vi "Main_19A.vi"() -> ()   [LabVIEW 2024]
uses:
  ENUM_Stripe Select.ctl
  Utility/Universal Utility/TypeDefs_Utility/Cluster_Row-Column.ctl
  9e3f57c0-2ef8-4495-8287-c6a42a5fb955.vi
  Utility/Universal Utility/TypeDefs_Utility/ENUM_4 Directions U-D-L-R.ctl
  Utility/Universal Utility/TypeDefs_Utility/ENUM_8 Directions U-D-L-R.ctl
panel:
  out "Array":cluster{"Numeric":i32, "Array":T1[]}[](array[cluster])
  out "string array 2":string[](array[string])
  out "string array":string[](array[string])
  in  "Select Data":enum32{"Example", "Puzzle"}(tab)
  in  "Example":string="r, wr, b, g, bwu, rb, gb, br\n\nbrwrr\nbggr\ngbbr\nrrbgbr\nubwu\nbwurrg\nbrgr\nbbrgwb"
  in  "Puzzle":string="wwubu, guw, uguggg, bgr, rgbrg, bbrb, rwgru, bwgr, uwwbuw, rwrbrgb, ggbrbuur, bb, ugu, grurrr, gbwbwb, rgbrb, bgrwrbu, bgb, wrwu, rwwr, wubr, bug, wu, brwu, w, grbw, uwbgg, gggwrggb, rurgr, uuw, bbw, wbg, bgw, ugw, brb, uww, buww, uuwgr, buu, rrbugw, ggggbgug, wwwrbbr, rgbbr, ugrr, wgwrg, bwuubub, uugg, bbrgg, bbugw, wuuwb, uwr, bugww, rwrrbbr, ugwrrrb, ubbr, rrwbgg, wb, wgr, gbrb, gwgg, rbg, bub, brg, bubr, ugggw, uuugbbb, grbug, rbww, rg, wgwwwwg, wgb, brugbbb, wgrww, bbrgrurg, ruu, brr, grgwg, wurbb, bww, ubwgr, bburwurb, urrrrbb, rgg, wwww, gbgw, rbrb, buw, wur, ruugugb, uwugg, rgrrugub, ggg, ggr, wrurr, bgg, uuru, brbg, rrbb, bbr, gbbu, grug, rwrrug, ggubub, ggrgg, uu, grb, rrrwwbg, ubbg, wgwwrgbr, rbug, rwrgwbrb, wubwgu, rrw, ruw, rbwubwgr, wwugg, bbbu, wgwr, rwgb, ruwg, rrrb, ubw, rwgw, wbr, uwgrb, rbwrrrru, guwbwg, rgbwr, wbu, ubgu, uruug, urbuuruw, rug, wg, gugbw, brw, wgrb, rbwu, wrw, bgggr, rubu, ur, uggrur, ggwbbuwu, gggr, gwu, bbwb, rrru, rubgb, wub, rgb, rbur, wuwbb, rbb, bwb, wwr, wubrwb, bwwwg, wwbwww, ugrrurw, grg, gwuw, uwwww, ubgb, gwr, gwuurgg, grwuu, gbru, rbbrrg, r, rgbrrg, ugrrubr, bw, wwbwbg, brbwbwr, rrrbg, rggb, bgwu, rrgrwwb, wrgrrb, grw, ubu, wgrugw, bbrugug, wubuwrb, gbrr, rrbg, bbg, bgrwg, urwu, uug, gruruwb, bur, rbwrguw, gbbuw, wubbr, gwurrw, rurr, gwrubb, wwwrw, wrwrbbr, ubbru, gbr, rwg, rrgwgr, ugrwwg, wwbgbr, wwubuwu, uwbb, gggbb, bru, uwb, bgru, wgu, gbrgr, urrwb, ub, u, bgrug, rrwr, bguug, gwbb, uuu, brubwg, bwrwbu, ruggur, gggww, rgu, ug, gur, wgurgwb, uuwwb, wbwgr, gbrg, rru, uuwurrr, rbgbw, ubgwgw, wgwbgu, brbwgg, uwwgw, rgww, buuu, uwu, wrgug, gug, rr, gggwb, bgu, grwg, wrwr, uub, gbuwwrwr, bgug, bwg, ubg, urrb, bbgggw, uuurb, ggw, wgrbwrg, bguw, brrrb, gwrbr, brbw, ggrrbu, uru, wrrbg, ubr, ggrr, ww, wwbgwwr, bgrr, wugbrwg, rrrrg, rww, wrbg, ubur, gwb, rgw, bubgbw, gbb, buuuuur, wwu, uubwww, buwg, ugbg, wgrwbub, wurwuu, bbu, wuru, ggu, wguwgr, gbw, gub, grr, rubgw, urrurb, wbubrr, grgwwb, gbwwru, urb, ruuw, urr, gu, bwrbwg, wrr, wru, wug, wbuwwwwg, guugu, brwurrb, brruuw, wuuuu, rbu, gwg, bgwg, rgr, bbrw, bu, gbbg, bbub, bwr, buur, wrgg, wwuurbug, bgbu, ruburubr, bwurbr, rbr, wgw, gwwug, rruu, wubgg, bwwg, wgwbwu, gwrr, wbbrrb, rwbgbbbr, gr, rwuw, rggbur, gbu, uggb, gwgr, guggbuu, gugw, brgww, wuw, rbubgbu, wgwbrb, g, urbb, gb, gbwu, uuug, ggrbbw, wbrrww, wbw, ugb, gbg, ugr, ggwww, rwr, rbrbw, wrg, wwbr, uggu, rrg, gwguuuuu, bbwuur, rgru, bburww, bbbg, wbb, uuugww, bwgg, bgggw, rugbr, wugrbwr, urw, bwu, uur, gggwrw, buwr, rrr, wwb, wgbw, urg, uwgbw, gru, bgbgurw, rwrrgbub, rwrw, buuug, wggbrgw, guu, bruuubw, gw, wuu, rrb, uuuwg, uwbugu, ugbbrr, wr, uw, ruwbw, wwg, ubru, guub, wrrwg, www, bbuuuw, guruub, wwbrwu, rwgbuu, rguruww, bgggrwr, bg, uwuwr, ugwub, ubgbu, ubbur, rub, gww, rw, urrbbbbu, urrbb, wuwu, ubuggww, bbbwg, ubugg, grgb, rwu, rugbug, ugg, wgg, gg, ru, wruw, wrrwuw, rubg, rbw, rwgwr, uuruu, ubb, ggb\n\nuwgwguuguruwggwbrbwurruwgwwwurgbgwggwwbbubgugguuurgugugwu\ngwwggrgbwbbguwgbguubbwrbgurgbburrgbwruwgurgwgguwbwgbgrr\nrgggbwgwgwuubwbwrrbrrrurwuwurgubuwrbwrbbbbr\nrguruururrwbbrgrbgrbwggrubbggbrbrugrgugggurubrbuuw\nrruggbrruruggubguwrubwbwuwgrwrguuurbrrbbbggbrwg\nwbwurbbrggubugbrgrrbuuwubwurrwururgbgbwurubbuuwbuw\nbrbwrrruwrrrubrwuugrbuuwuuwrwrbrrgububwurugbwwrb\nrbbbuurubwubbuguggrgwgwgurburugugwbgbuwbwwrrgugg\nwrbbugrwgwubgugwrruggwwggurrwuugrwrwbrwgrww\ngbwbugwgrubbbbburrbwugbwuugrbbwrrwbgrwubgwgbbb\nurgrwbruurbbururwrwwbbubgwbwurbwguguwgrbrgugugwrburb\nwubuubwggrgwgbgububrwgwbbubgwgbwwwuubrbbbuwbr\nwrrrrurbwubwuuggwguuwwwububrwrruwurrbbbuubggwgrgwugwu\nbrurwwrbbuwgugbruurgrrgbuuwrbwrugurrwrurrrbbwrwbrrgrwuwg\nurgwuwwbwwrbbwbwgwgrrbrwgubbrbgwububbwurggbrgrggbrggrrrwgg\nuugwrbwguuwwgbwwwburburbwburwgwguwggwggwbbbuburrubgbbguugg\nwbwbguuuuubwwbwgrwbwgguguwgbbggwwwurgrwgrgbgggurbuwugwrbu\nuubwuwuuwggbbruwuwbwbgwbwrrguwurubbguwwgbug\nbwwgwwubbrrrrwuubwbwrruurrwwwwggbgbrwububwwurbggwuwbgu\nbruwgrwwbrwbgruubwbbbugwrbbgwguuwguurbrwrb\ngrbgwuwwrbgrwgrwurrwbbuwwwwwbrbburrbrwbuggrgwbwrb\nwgggrubbbwwgwgggwruururugbrguburrwuwwurgggubrbwwgrwrb\nwurbwrwwugrgrgruruuggbbggubwrurbrgrbwwrbrrw\nuubuwwurrrrurubbbrrugugubgbruubbrwbuwugrwwgwrrbrwggwrb\nggbuwrwwwbbrgruugrrbrbuurwgurwgubrggguwbubrrbbwgwrb\nugwgurwrwwbrrbwrrrruwbgrwrurrrrrgugurwbuuubbubwwbgrrrbwrb\nurwrbbrbwgurbuwrgrurgwggubbwubuggrgbuwgurbbwwbbwwubwrurgrw\nbbugbwrwrrrwbgugbgguuwwbrwbbwgurubrgugrgwurrbb\nuburggbrbuurrbbggububwbuuubgwrruugbrrbuuwb\nrrwuwubggwrwruwrgrrwrwubwwrbbbuggbrggurubwubwbuggwu\nrwwuuubguwgwuwgwwwggwbwrubbrguuubrurbwuggubwbruwrb\nruugbuurwwwwrwuwurrrbrubugubwrwwwgbwbrbgbwb\nwrurbuuruwrbwgrbgbbwgwrwrrrwgwrurbrbuwrwwgbgwgrwgu\nbbruguugubrrgrgurwwggwurwbgwbwbbuugwwrbwubwgrwrb\nbbwgrrugwgrbgwbbugugwuubrbrbrbbrrrggurgbbwwuwrbbuwbgw\nrbgbwburggggrbwubbrrrrggbuwbguggrrbuwbgugbbrgwrb\nubgwuwbbgbubrgbububwuwbbbburwurbwbbuburwrb\nbbgubwgruwbuwbwrwrurbrbrubuwbgrugwbbggbwgrwrburguggwwg\nuwuubwuwgbuurbugubbgguburbugugrrwbrrurgwrwgrgbb\nwwuuugrwuwurbgwwbrbwguwugbgrbgwwbgrgbubrrgrbbgwrggwgrwgruu\nbbbwurgwwbwurwubbugrwbwbgbwrbwrwububbgbgurwwruwrwrrggrugr\nbubuwbbwrgrwuggbgrgwbbwruubggubuwguwgrbrrguwgwubbbbubugw\nwbwbguwgbrgwgwrrurwwrrrgbrwubrgwbwguwbwwuwgugwgrbbubgru\nbwbrbwbrbubbwwbgwwuwgwwgggrrgwbubbubwwwugrgwgr\nwgwwwwurwubuugruwbrrguwgubwwbuuwruugbwrubr\nrgbbbwrgburwuwwbwubwruubgguwbrbwbwrwurbggbwbrugwgrubrgbbur\ngguwwggubgrgrgrwuubruuurubrbrruwgrrwrwuwgrwwburwuwrg\nuwbgrrwbbggrwwgguwbbgbbrugruugbgrbuwgbugwrb\nguurgurbwbbrugrbuugbgruwgburwrwwrbgbrrrgbwbuwrb\nuuwuggwrwgbgbuguruwrgbrbrubgrgugwbrugwrgubbrwuwrb\nrwgguuubwrbbrbubbgwwgrgbbrrrgggbururgwgbwgugwgbgbrbbb\ngrwwrwbbruwubgbwuuubwgubguruugubbwggrgurrbwurgubbggwb\nbwuwbggbwbgwbruuggruurrwrwgubbwrrubrwwbgubguwrb\nrbwbbrgrwgbgwgbwrrurgbrwgwurrwbrwwuwrgugrbgrugrgubbwrb\nwbbgwgbwrubuwgurwbwbugwguwwwgbuwgruguwbgbgbuubwuwgwubgrbww\nuwwbwrbubgbwwuwwubbgbgubwwwgwugrgugrwwwgwbubrguggbrgrbrgg\nwbwuwgrwwguwgurwwurwubgwuwugrbbggbrruuwbgurrru\ngbugwgrurugwrrggbrbubrugggwggbubwbwrubububgbwrgwuurugwrb\ngugrgwugubwuwbbbuurrwwrubbwwwguguwwbbruuugbrwwwuwuw\nrwbbgbugrgburrggrgwgubggwwruuggubururggrbwrb\nrgggggrbbrgrrugwwwgwbwbbrrbrburbwbwwrrgrbuugrruwbbuwrb\nubbuurgrwwwuwbwwbgguurbbbgwbuugwgwuggrrbugguruwwrgbgggbbuwrb\nbwuruwwubgubbggrruwgbbgggwrruubgurbrbuuubrgbwub\nrbubbggrbwbgwwrrbbggubwwurwgrgwubgrgrrbwrb\ngwwbgwubrububgwrurwgurbbuuubwugggbrrwuuwru\nwguggrbbbwgrbrwwggrurwbggwgbrgggrwggugbrgwgg\nuuguuwwrguwrrggugbwwgwuwrguwbguwuurbwbwrggwguwrubwrb\nruuubbgrgrrrgbbrbgbrbubgbubwguububuugubgrugbgrgwrgwrwruggw\nruurrbwrbgubbuwggguwbwububrbwgrubbwgugwrb\nbbgbugbrubwggbrrwwuwrwwwwrwbgbbggrrwbguwrbwrb\nbrbugwrwrbwwwguwrgrrrggugwwruwburugurrgrurbguwguwwbrubu\nwbwubgbubwwgrrggrbbgwruwrrugwwrwuuggbuuwburbrugbguwrwrb\nuugbuuwwburgbgruuruguuuwrbwurwggbbwrrbgrurbwub\ngrrwguwurwwuwgguuugurwrgurrwgrgugrurururwrb\nwwrbuwwwwrbbgwgwbgrurburbbwbgwuugbuwuuwwuuwbbuww\ngggrbrwrugrrurwugwgbgugrruwrrruurbwuubbuuruuub\nrwuguwurugbrububbrggrwrwururwuwuwbrwwgurwgrrrrbrururrwbgbwrb\nrwbbgrbbwgbrbbgugggwwububugrbrgwgubbggwgrgrbrrbrgwwuwg\nwururwgrruuwrgrrrwbruubuuwgbrrwbgrrbbbgugbgrrguugwg\nuruwurbgrwrgwbrbbggwwbgwbgwrbrgrrugwbwrwwbggbrgrugwrb\nwrubuwbugurguuurugburubbrgrurgwugwwbbwuwrb\nbwrwgbwwbuuwbwgbwbbbrbwgwrugbubbgubuwrrwguurgrurwwwbwrb\nrrwuuwbruwugwguurgubwrgwgwgburbrwwwgbubwrwrgggrwugurbrrbu\nrrwgrgwwubwgwbrubwurbbrgbuguwbuggbrwrururrubbwburw\nuubrgrrbgguggwrbwbwwwguwugugbbuubgugrrbugbruggrwubu\nuwrrubgbrrgrbgrrrgbrwgwgrwbwgugguwwwgruwbuwwrb\nwbgubgrbrrrwbgrbrwrggugruuguugubbwrrwugbbrubrrbuubbwrbwrgw\ngubggguubrrguwrwurubwwubbugrwugwugguugguugbuwwwwubgwgbwwuu\ngwguwggwgwbrugwbgbgruwbrwgbgrwbgubbbgwgwbggrw\nwwwburgwwurgubugwrubrggbgbrrbgbwgggwrggbwbbbbubrbuuw\ngggggubgburbgrguurbruuruguwubrrrbruruuguwwwgggu\nbggruubuugbbubugwrrbuuwrguggrwrwurubgbwwwbuuuwgubguruw\ngwgbrgburrbbgrwgrurguuwrrwgggrbgbbgwbbbwrgggwbrbrgwur\nwbbbbrggurwuugbruubrbwgwgurbwuwbrbwrbwgruwrwwgrwurwuruwrb\nbbggrguugwrguwbgruwrwbggurbguuuubgrurwbbgurrbgguggubw\nuwrrwbwubbgwbuwwuwurgwurbrruruwuwguggrwbwwurwwurgbgu\nubuubuwrgrwugguuubwwgwrruwwbuwggbbwwrrwbrgbuugugwwr\nrwwbbugwrwggwwwuwwbgwwrrrbggruruburubrrubggrgwrb\nbbgbrwgwrgguwwrubgwbgubuuurbwwbbbbuggbrgbwrb\nubugbuwbrguwwbrgwrgguwwburgbuubwwgbgrbrubgbgr\nrubwrrgurbuwbrggwgbgwbggwuwrbuwgbgubrrrgrrwgbbg\nubrbrrgurwbgbbbrrrugbrwwgwugbrgbugugugrbbggrwbgubbbuuub\nwuwgububguurguugwuwbuwubgruwbwuwbubuwburbgg\nwwrbgwrgwubwrgruuggwbwwbrbggurburgrggubgwrrgrgrgbbrbgwwuuwrb\ngbgrrbugugwrrbuwrubwuwwgggwrbwwrugbgbgrgrrruw\nbwwgwruwugwrgwwburrwrgwgubbrgurgubrwwrggrggbwwgrguuwww\nrbbwurrgrwrbuwruwuwuuwrgugbwrgrgruubwburbrgbrubgrgrwguur\ngwwuurbugbgwuggwwwwwbwgrrbbgrgwwbwgrggrwrbugwrwrb\nugwrbrgrggwbwwuubrwubuuwwurbbbbwgggwgurbggw\nbbwggbubgwwuurbuguruwwbgggurgwbgrgrggwurrrrurgbrrugrgwgww\nuugwuwubrurururbggrrgurwgwgrrgwwgrwurwrwurwgruu\nuwgbwurruruwwuwgbbgwwrrwrwbwgrrbwbrwgwbbwubrgruwub\nguugbrrubwbrbgwrwwrurrwwgbbgwgwrbuggurgruuwgrub\ngbgurwuuwubrrugwrrugwbbbrwbrwuggrwrrugrwbgu\nbwguugwwwuruguwrrwwbbuguugbggbwbubbwgwrgbbguguruwguwuru\nbbwrbrguwrwbrgruguuggbgrbrruguubbuwwgrbbuwrwwgrbwb\nbuwbwbbrurrbubrwgrgwwwbgburbruruwbbbubwrbuuwgwwbwu\nurgrrrurgwrggugwbrwubgguguuruurubbwrrrwrb\nbburwruuwbugrbwruuuwguubrbuwuwbgbgrbubuwbgr\nrbgrugguurbrrbbwruuuuwgwrggwwurbbrggwrruuuurgggbrbrbrb\nrguwurugbwbwrbbggrgbgrgbwwuwrbbubugrwrgrrrbbbrburgubgurggwrb\ngwuwuuwugwgguubruwwrubrurwrgwrbbgruuuubwwurrugwuuugwubg\nbgubgwwbrbrwruugbbbbbwrbguwbgwgubgbbgbbgurgrurgggugbbwbr\ngruwwbwwgbbwwbwgwgwwubwwbwubwrwrgurwuwgrbbrurgwg\nguguwggbbbgbggbrbrgwbgbrwbgrgruurwurbwggbuwug\nrbrbbuurgbgbgbgggbrrwuwuwgwbwbwwuwbgubbbbwr\nbgbuwugbugrwwwwgrbbgguwbrbwuuwgrgggrrbgwbwgruggggwwubbwrb\nggwuurgbwurbwubbrgbbubgrwguwbrwbrruwgwgbrwgrrurggwub\ngggruuubuwrrugggruuguubbrbbgbruubuwrurwbrwggbrgrrburwggw\nrrugwrwbrgbbwrgwgbbbrwrgbburubggugrwggrbrbwubrgurgbwrb\ngrbrubguwruuwggbwugwwgwuwwggubuwuwwrggbrbuurwubwbbwrb\nuwbwuwwbbrguburrwrugburgrwuruwugbburubwguugwwru\nuuwwrubggwwwuugrgwbwgbbwrrbburuguurbrbwuwwrbggurbbwguuw\nubugbwrguwrrwurwuwbrbbubbbwbgugwgbrbwruwwwrububgur\nggrrburgrgburuwrrubububrrbgruuguuuwwwgwwrgbruub\nggbuugwurgbgrwggurugubwggbbbubrgurrwwburuggrrrgbbbbwg\nggbrgrwuuwwbwbuwwwwgguwbbuwuwuwuwrwgwwubwwuwrb\nwrbrgugwrbwrwguggrrggbguwrguuwbwwrrubgbbbuwwrrbrg\ngbwbwrgrbwurwuggwwrwwgwrbbwrwwrbrrrrbuwuurrburruu\nbgugggbbburbbbrguurbgrugwwgggurugbuubuugubwrwr\nwrgbrrrbwwurbgbgbwbuuwbwwbugbgbugrwgwuuubugwrggwwbbbwggwgwrb\nwwbwbbrwrbruwrurwurwggwwbrbuugbugbrwgubggrr\nbrbubbburuwgrbuwwuwrurrwwubrwugwbgburgwrggbwuwrguwgwuu\nrwurrbrggrrgbbgbuububrrwbguwrgbwruwgrrruburuurwwrwbuwgbbr\nbwggbuggrwuubrrwubuwrgwrbuwwurugrbbguuwrrugbgburggububww\ngruuwburbbgbrbwgugwgwuurgububuwugguwuwwrbw\ngrrbgwbwrbrwgwrwuugwbbgrrggggwuwgwugbbgugwbrugwbwu\nrugruggwruburugwugrgwbugwwugwuwrrgrgrggubrgbwgwwwg\nurubrbgbgrgwwgwbrgbbwbrruuruuruuururggubwr\nburbwguggwrggrwggubuurrgwbgwggwrugwwuubgrbwbgrrbug\nwwbwgrrwbwwbrugrbgwgwgrwwggwbrbwbgggguuubwbgbburguggub\nurrbbbburgwbwbbwrgubbggrwbbubuwrgggubggwrb\nggugrbggurrbggrwruwgrbrwgwbuurrgrwwwgugurrrbwgbbrbbggwrb\nbwgubwruwrgbrbwgbwbbgbwbgrbbruubbuugwburwrb\ngwrbbrwugurrbugrbgruwruwrwwguwubwubwbrwgrruggrr\nrwgubrrugrwwwubrwwwrbrwwrbgruwgrubbgwgrwrb\nbrrbwgwgwggugbgrrrrgggubbwwwuururbgbrwugwbrbrbwuuwru\nurbrurgrbgguguguuruwurgugwwgrubggbgbwwwgrbugubwggr\nrbgruguwrurwbgwgurrwrrrggugrwwbrbrbwgubuwubruubwrurrgwbgbwrb\nggbwuuuwggggrububwwrurgbrbrubbwgbbbgbbbgbwuwwgggbwrbuwrb\nrbbbburwggwurrrrbggwgwwrurubwbgbrbruguwwrwrgggrugubw\nrgwgwwrgbrgrwgrrbrburwbwuugbgrwwwggrwrbbwrb\nubgrwwwuubwwwwgbbrurbuuruuurrbuwggbbuurgrrwrgwb\nwgwwuruurbgwruugrwgrbugrbbwbgwwgguubrwrrbr\nbwrwubggwgrrubgrrwuwuuugruuuubuwbrbbwrrbgrwugwgwugrguwrb\nrguwgwugururbwwgwwwgwgwbugubbrbrgwrwgguguwbwruwrrrbgbu\nwuuuugurbwrgbuugbrrwgggwwwrwrrrrgwrwggwrbb\nwwbwbugrwbbuwwwrwrrrubrbgwwwburwgbgbwwbuwrwugguurbg\nubgbuubgrrwruwugwbwbwbwwgbwbuurwwuwbubwrbug\nuubgrgrrugubggggwgrbgbrwrwbrgrwbbwgrburrbr\ngbwwugwbgggrbguurbrburbwwrugguwbugwwugbuwwbguu\nwuwgrgrgwgrbuwgrbgburuuwrbwguuwuruwgbwwubwwbururbw\nwwrwgugurwrbbbrwbwubggguuwrwbuurbwbwubggbbuurrwwbubuwrg\nbburgruburubrbwrwwwbrgrbuwgwrwggurburubrgwgbbruw\nubrwbwubbbbwbwgruwuuwbrgbuwwuwuurrrwrrrwgb\nwwwwrbrrguwugugbgrggrubbrgrurggbgbuwwbrgggwuguwugbrwg\nrbrbbuwrubbbugbgwgurggrgbwrrurbburwrwggruwrubgbgwwuuu\nwuuugbgwgggburrrrgwbubbbgrubbgburwrbugbbwbwggrgrg\nrugwgubuwurrguwbwwurrggrgrurgwbbwbubwwgbgrubruuuwwbu\nbgburwubrrwburrbwgwuwwwwurwuuwbgbgrwggubuwubwwggrwrb\nuurbururruggwrwuwbguwwwbbwrbbwrggwrgbwwugwrwuwrw\nbburugbugwwwwggggwruwwggrwwrbrrbwgbbbuwgwgbwwwubgrgbwrw\nrgggubrrbgugguwwuuwurgubgwrbuwubwburwuubrgb\nrwrgwbrbbwrbuwwuurgwuwwbrbrwuububrgubbrbwrguruuub\nuuugrguwruwwuwuuwgbbrrwwgruuwbbgwguwwruuwrb\nbubbubgwwuurgwrbuuurrwrwwrurwgbwugguwgbbggggww\nuwruwuguubrrbbggbgrbwrwwwbwwwggggruuuguuugbwrwwrgw\ngururwuubwbbugububgwugbugguwuwgwrugbrwrwrb\nwrrbwuuwbwbubgwrruwgguwgrbggubrgbgugrrgrubwwwbwbr\nrbgwbgwububrrrwbuwwwwgrurwrbwrgurwruggguggurrrubbbwrwgww\nwggbrggbrrgbrrgrggwbbwurbbrgugugrbrgrwwbrgubwrwuuruubwugwrb\nrrgbggurbrwuwrgrbbwwubguwgurugurwurwbgwrrbbwwuwwbg\nwbbggrwrgruwgrbrgburwggrrbbbguurgubbuwbruwwrggrbr\nwubugrwrrwuuugwuubgrubbbbgurguwgrwgruwwruguburwuwu\nwbwuggubbrwugwbwrrwurgubuurrrubrgwbruugrgbrrbrugbwrruwuubwrb\nrrbuwruwguburwgugrwgwuguwuubgurggrbuugbuwrb\nwrrbuwggurrggwubgwwuggbwuuwwurrrwwrwurrburgwbwugrgbuwwrwrb\ngrrurwggwgruwrrbbwuugrwgrgggbrgubggbugugrwrb\nwwwrwbuuwgbugbwurrgwuwbuuwrbuurugurwbuuuburrurwrb\nruruggbgwbggrwwrwrbrrgwuguwwrwurrguwugurbbruwbrwuu\nuwuuggwurgbwrrrbruwrrwrurgrwrbrwugrwbbburwurbwbru\nrrbwuwgrwuugwguugbrwgubrbubgguwrugrwbwrrbggbgrrrugrbbgr\nrgggrbugbubburuwwbrrrbuubrrwubuuuwgbgguuuurrubrwwuwwugrbwrb\nurrgwwwrgwrrgurrgwbbrggwrgubwgwwwugruuubuuwggbuur\ngbuguuwwrbggrwrrubwwgrbwrurugrwrguuuugwgwrrrgubgbwb\ngwugrrwrgubuwggwrrguubugwrbururwgbwgbbugwwwrb\nbruuwuwbgrbrwbwwubrbbwrgwubgggwugbuwgbrwbbwruubgwbbrwwwubg\nwwgurbbbbbwbwwrwguwbrururbwurgbgwurrurbgur\nwwrgwuurruwuwugbbrwbwrbbbuwgwwububrwwgggbguwrgwrwrrub\ngugwrrrwugugruuwrguwbwwubbggrwbgbwrugbuwrb\nrgubwgbggwbbwggwgggrrrgggbuwwrgrwggggrrgwr\ngbgrbggbgggggbgugwgubggwrwwwrwgrbrguwuwgwrbbrbuwwgrwuwrb\nwwbgrrggrbgrbwbrrrbwrwrwbwrbrrwbwuugggwrb\nwbbwbwbgrbwwwuguubbwgugrugbbrbbggrwwurururwggw\nuguwrggruugrgwwuubbrbbbgbbgugurruwruwbugwrugubwwbgbwg\nruwbwbrubggruwbrwrurbrrrbgrrwrrgbubbrwrwurwuubwbrruburwuwrb\nugrrbgbbugruruwbgbbbgwbuwgbwugurbrwbgurggbubwwrbb\nwbbwrwrwgurubwgbrgwgrgggrguruubburrubwugggrrwgbbrugw\nuugwubrgwuuwbrrrbgruuwruwwbuuubgwuwwwuwbruguuuwgrbrwrb\ngugubrrggwbuugubrbgwgbubwwgrrurubwwrbbwbrgrr\nwrggwguuguuwbgburwwgwgwbruwrgrrwuwwrgbgugurwggbbg\nwwuugbgggubwwwgrgrbguguwgwwwgbuwgbugwgwwguwrug\nuwuurugbwgbrrbgbbuuwuggbrbrwubwbrggwbgrubbrrggbuubu\ngwggubgwgubguwrbggbwwgbuurbbuubuwwugbubwbgbbruu\nbbubugbuwwgbgubrbrguwggbbugggbuwuubbwgrwgwg\nrrrrwugwuurrrbggrbwbrbrugbrbubugrbubbrguwwwwwrrgwgbuugbu\nwrurguruugbwrwbgguggbwruwgbbwgguurwbgubwruuwru\nrwbbwbrbwuwrubgbgwrbbuwbgubrgbwrrwwuwgbrwgurgubburuug\nggwubrwwuggrrwbuuubwwgbbgwurwgrgwwuwubbrgruurugwuguggurg\nbbrugurbrurbgrbubwurrubbrbbgugwbbbwuuuwrb\nwwgwwbruuuruwggbbwuuuubgwbubrbgwbwwuruuguw\ngburwbwbgrbwbgrugbuwubgrrbrrggbuwwrwrwbguuuu\nuwuwgrbggbrwgwggwwgbrrwburuuguwbbwwwrgurbgurrwgwurguwrbwu\nrbwrbuwrwgbbwwggrbwbwwggrwguwggbwrgbrrubgubgugwbrruwwrb\nbbuggbgbwgwrrrggbubrggrurugubuwbwuguwbugrrggwuwbwrggbwb\nugggrbwgwuubwwggggwuwwwruuugrrguwwbwubrrwugwrrurwgbg\nbwgrgbubgbuurggguubwwrwgbubgrrgrgugwrguwruwbrbwrwbbwbbbb\nwrrrbgrbggruggbbuwwuubrruwgbuuubgwbguurrubbubb\nrbwrrrrubruuwgrgrbgwwwurwurgwbugrbbwwgggugbu\nugbggrgrguwwwggbruuruubwwgbwuggwbrwbwwbrbwubrubgbrrgwuwrwrb\nrwrbrubwbburrurbuwgrrrgurwgrwbrgwgwwrbwgbrwr\nwbwrbruubggrgwbbrbgrbuwwrrrbwwburwgwguubuwguwbrgubbwrbrbwrb\nrgrrbwrgwbbuuuruuwbrubbbuburguuburrbgrwbgruwru\ngwrgrrbubrwgurwgruwguurgruruubgubguggbbwwrb\nwgbbuwurburbwwurgbgbwgggruggwurbwuwbubrwrrwbburbgrwgug\nubugbggwuwguwwwuwugwbwgwwuuuggrrrrubwwubwbwrwrrugwbwrgwuu\nrubggguguuwgbuwggrruwrwrgruruguurrubwuwrgruwwgrrurbwuw\nwurbburwrubbwbwrruwrbrbuuugurbwuwwgrbrbggwwbgugubrrg\ngugruugwruwuwrugbgurguguuwwbbrwrurrgubwbwbrgbwrb\nwugrbrbgwbbuuwrrgrbwgwrruuuubrbruwggurgbrg\nrurwugugguurgubwbuuuurrrwbrrurbwruurwugrubrgubwrub\nrubgwwrrwwwgguuggbwuruwwggbrubwbrwgubrrgrwwbuwggbbburwurbwrb\nwbbbggwuwbwwgguruwguwbugwgruwwrwrgggurwwuwbbwubgu\nbgbwbbwruuugugbrwburuwwrwbbbuggugbwubrrwgwugbwguguuuwru\nrbrwwwwwgbruwguuuuubruuurgbuubrwbrbrwurgburbub\ngrruruwbrwwrbgrgbgrwuwrgwwuwbbwgrrrrrrrrrggbbbwbbbbu\nurrwbbbrwuggrggbgububbrbubuwggwuugwurbbbwbbrwrb\nrwwubggwrrbuurwwrrruuuruwggggwbbuwurrurugg\nbgrbrruwrrgrwbwruwbwbguugbrrggrbgububwbuubrububggugg\nrwruuwbuwruuwrrwgbwwrbwwwbwwrwwuuggbggwbbrbbbwwg\nrrgwrgwubgwrwugbuurgruburburuwwwbwwwwrgwwrgwrgrgg\nwgwrrgwwurrrubwgwrgbrbwgbbubrrrgugwwguubuwrbbb\ngurggwuurwwurwrggugwugrbwubggwwwugrbubwrubbuw\nuruuwurrggwbgrugrrbbubwbwwggbuuugwgrwbuuuugrrwbr\nwbbguguuwuubwwrbrbbrugwrwuuwgrggbbwurrubrrgwwrb\nrruuugbgbgrrwwrwgrbugburbubuuggurguugbwgggwrwwbubb\nbrbgwwbgrugurrgurbbwbrwubbrbrrwugwrwugrwwrb\nbuurubwuubrwbugwbbrrgwbgubrggubwurggwbrwwrrurubwrgrrg\nwbrbrrrgrrbwubwgrwubgrgrwuubbgwwwugbwruwugwwgubww\nuwrgbrubwbuubuurrrbwuguwbggurbubuwgwbwrggbggbwruwuggguwbw\ngwbwgbwbgrwbgbbbrwwggbgrurgrwguwgrbruuwbugwrbuwwbwrb\nguwbwbrwgbgrrrbbrbruwwbbuwwggbwrrbuubugwbrwrb\nwrubrurubbbuguurrbguugwurwuuuwgubrwbbgguwwbbbwwwrbwgwuwgr\nrurgbrrbwwbgwbubuggwugrubbgwwwrubuuwbgwgbgwugrrugrub\nrwugwrwwbuggwbugbbwrbwwruggbgrwuugruurgrbwwbuwwurubgbr\nbwbwuuubbgurgrgrbggrubuuwrugwgwuwggwrggbrbwubwgwguwwrb\nurrgurwuwwggrubgrrwrugbbgbbbgwrguggrbuggrgrgwrb\nwuwurrrrwbwgwwggurwuwbrrgrburggbwgrggbgrbrrggburrggwwrb\nubugrbugubbwgbbbwwgwgwgbguwwbrgbrgwubbwgwwruubgrgrrrb\ngurwwrggbbbburwbgububbrwrggbuwgbwrbrrugburgrgbu\nubgbbrrbubrrubbggrbgwbwrbrwubwuurgwbburwwgr\ngwbrrgwgubbbbrrubwgrguguggwwrbggrwrwuuururwrwguwgrbuwbuuwrb\nggbubbbbwruuggrwwuuwbbwubgbururrggrbbwgwrb\nrgbbrgrwgrruwrwbuurgugbrububrugbgwruwbrurbrwwuwbbrgbbrugr\nurruuurggrwgugbgrwgubrbbbbwuwrrwgrubrurgrbuwrgwu\nbbwwwwrbbuwubgrrgurbbruwrbrwguwrbwrurwwwbbuwgruubwwwrb\nrbrggubbuwguwbggbrrbbwrrurrrbuuuggugububbbbwrrwb\nugwgwwwrwruugwrwrbuggwuuwgbubwgrbrwwgrggrrgrbrbgbbwgwrb\nggugburbbrgrrwgwbwbwruuwugrbrrrurgwrbrrbrwubr\nububbrggggrbruugrubrwrbgbwggwrbrwubggubgggrrgbubrrgrwrb\nrrgwwwrugrurwuggggwrbbwugwwwwububgbrbguwwwguwguwrb\nuuwwwrbgrrbwgwuwrwwwgwwwrbbrbuggwwuguurwgwrb\ngurrrubbgwubwuggrrwwbbubbrgbgubruwrgubggrwgrburrrrg\nuwugubuuwurruwruubgbgbwwggbrwgwgrbbuwugwrb\nwwwrbwrbwwgbrbrwbrggrgwrurrbrbwuruuburbubguwwugggrbwgwgb\nwbgugurgwrrbbwugwbrwuwrwruruwrrugrruugwuggggw\nrwbrwwgrgwwgrwgwbgwrwrwguubuwwbguwggubwggwwbww\nrggrruwggwrrgggbrruwrgbuggbbgbwbwgurwrugwbgwwwr\ngbbwrgwwrwgguurbggrbgbwggbbbuuwururrgrgwgbgg\nwbgruwwwubrbugwbuwuubwgrubguwgwbrubrgwwwgwbgwwrrugbgbub\nugbwugubwgwbuggrurguwwubwrrurrbrgurrbrubwuwrwwwwwgwwgrwwbw\nwrwubuguggbrrbugwbwwwrguuuguubwuruugwbgwbguurgwwbggrwwbuwrb\nuuugbgrgwrugwguuuuurwgggrburwwgbwrurwbgrrwrb\nwbgwguuwbbuwggubrrwbgrgbwuwrgbubruwggbrrubbwg\nubuwbrwbbbwbguuwgugrbuwwrgugwubgrburbgbbrrgrubbbbbu\nugbubrurbgwgwwgrurbwugbwwwbbgbugbbbuggrwgrbugbgwwbuwrbuwrb\nwgrwwuugurbgrrgwwbwrubrgrrwwubgbuggwbbuwubu\ngbuwrwbrrrwrwbwwrgbugrbugbrurrgggrgwgwgrrbgubrr\nwugbuggubuggbrggubwgggbgbgbgurrgwwbrwwwwrb\ngrgugwubbugurgbguwbgbrugwbugbrrwubwrwuwrgbrugrgwrwrb\nguruwwrurwurwugbbrbwwwwubuwrwuuwwugwruwbggbbb\nbguruwbbggggbgugrbgrrrgubbbrubwrrwrwubrwgrurw\nwbbrbbrgbbgguwbruuguwbbbrbrgrubgugwrgbrrgrwruguwrb\nwgrbrgbrgwurggggurwwwggubbggrrrgrubugwuggb\nbbwuwwrwrrubruuggwwbrurbgwururwggwwrrrurrww\nubwuugrgwuuuwururbrguurgrbwwwrrwbwruwrgwururbugrwrru\nrgbbrwbbguggwbrwwbbgrburwbbwwgbrbwbbubwwrb\nuuwuuubgurwwggwwbbbgbgbwbrrgbrrwrbbuwwwgubgggbbrwbrr\ngbuurwggrrggbbrgbuuwrgrggrwgwwrwugugwbgwwbrr\nbwbrgwbrgwwubrgubbbuwbrubwrbgbrrbbbbwrwbgwguuuuubrgrgrw\nguwguururgwuwuuwgwbruguwbbubuwbrggwwugrwruruuugrwrb\ngrgwuuwrbbgrrgggbwrugbgwbbbrwuuwuwgbwugwruurrrbbuggrwwwru\nbuwggggwrrrruburwbrugrwrrgwuguwggwbwbgugrgugwwurbbburrggw\nugrwgbbwwwbbgruubgguuruuuururwwbuugbgwwrgubrrbuwwugggw\nwbrbbugwgburbgrbgrurrbwwwrbwbwubbgrurrurwwrrbwgbugugw\nugugwbwwgrrgrgbuubwrwbrrurrgbubggwrgbugwrgbggubbruubgw\nbwwubbgwwrrwruuruguugugrwgwubbguburuurwguwbwrwrb\nbrrbwugubgwrgurrrgrbbrwrurugrugwuggwrgrbrwggwbbuwurrwwruwrb\nrwbbrbgwgbwguwgbgwurgrbuurugrrgwuwuurubrbgr\nuwwbuuwgbwgggwrububuugrwurgggwgbwbubuurgbwrrwbbrwuruwrrrb\nbbgwbwrrruurwwugbggbbguggguurrbbbbuubbwbwrwbrwurrbuwgrb\ngwgwbwgguwwrwugugwuuwurwgwgbuwgbgbwwuurwwggrubb\nrgburwwwuurrgbuwrgwrbugwwgguwwwgbubuuggrwbgubrwrgwugwbuwb\ngurrbwgburruggbrbuguugbguruwurbuugbrgbguguuuubwggrwgrrwbwwrb\nruggwuwgbgguwwuburgruwrbgbubbwwugrbwuwwbrbrrwbg\nwwbrrgguwbbguubbuuuuugwbbrwrrgrruwrgwwrbbbbwgrgw\nbwbrwbwwrwwuugugugbrbrbrrbwrwrruguwuwwubbugwgurrr\nwggrwwubuwruwgugrguggugwbbggugruuggrwbggrwbbw\ngbgubgbwgurbwrrrgbuwwguwrrwwbwuwuwbgburrbgwbgwr\ngrrububuwruwrubrgwwbrrgrbwugrggwbrgbwwrb\nuguuggrrwubrgrwggububbwgbbwgrwurwwwgwbubbbruggrwbrbgwrb\nbrgurrbwwugubrrgurrbbrbuubbwwwwguwwgrwwugubgruruu\nwrwubrrwburuwbrgwwuggurwrrwbbruruuwuwuwubbubuuu\nbwbugbrrbwugbwrubuwbuwwubbbguwbrgwwurbgugrgrwgwuwwbwubgwrwrb\nbwguwgurgurrrbgbbbwbrrrwuwbrwubruuwrbwrb\nrbubgwbubuwwbubbrgwwgubgwwrrgbubrwbbrwwrbwwuwgbbwrb\nwrbbgwburwwwrgwggggrrbubbggrbgbggwurwruburwubrubrgr\nrggurrwwgururrgrwwwgrugwwbguurbbwbuwrwurrrbrggbbbbrwwr\nugwwgwrgrgugrbbbbubrwrubrbguwbrwubgrwgrrgbgggwugw\nuwgrgbugbwbbggrgrbbgrwrbggrrwbbwbugwrwbrrwwuuwrb\nbguubugwggwguuggbguuwbgwbwruggwrbgbrrbwbrrbgwrbggwrbrrbu\nrgwwbubbbbuugubwbrwuwwrrruuwggrbbrbwguwruuubgbwwgwurbgbubg\nuuwbwbrwwubbrwuuuwuwwgggwwubburgwgwbrurrwbrbgbbburwgb\nwwrrbbwwbruwbgbggbrbbgrugubggwgggugrbuurgrbbgbuwu\nugrbwbwwgggwrgbbguugrgggwrggbuuwuwubrgbruwbwrb\nubggwbwguugbbubbgbbguubwuubrbwubrubrwguwwwrb\nrugburrbwruuwrwwgwrwggrubgwbuuubugbwuurgbg\nggrwrruwggbubrurubgwrbwrgbwgwuwrbbbwbuugwubrubwuwbrbgbgubg\ngrgwugwuwbgwuuwuugrgwwguwbburuubbbgubbuwgwg\nruwrwrwwrwgwwrgbubgbrbrwwbgurrwrrgbruuwgrgrrrgurugugu\nbrbwrgurrwgwrruwubrwwwrggbuururgrguwggwbbgrgubrw\nbbuwggrbugbbgbguugwuuwuubgwgbbrgugbgbwbrubbbgugwrgrgrgruuwrb\nwgbgbubuwrurbuuwgrugwrgrbrwrgwuwbbgwrrrrwrb\nwgwrgbbbuurubgwwrgwguururrubgbgwrbgwwwwwggggbrurgrr\nuwggrggrbrruwuruwbuwurrrwwwwbuggbguwuubwuwbubrrwrb\nugubbwurwurgwwrburwuugrurguuwruwwrwbgruggwbwwwgwbb\nubwgwbbgbrugguwrggubbrgrbgruuwugbgruuwggrbgwugugwugrrwwg\nwggrgugugubgrrrbugbbbwrrrwbwguuruugrwwrb\nbwgwwbrwbbubgwubrwwwgurbwbrwbubgbwbubwgbbggrrwbbgbwrbbrr\ngurwrbbbrbrurbrrbugrrrguurwwbbwugwbubuwrwbrgbgrwrbuuwrbuuw\ngwwwwuuubuguwwurubwwrggguwgbrbbbgbububgwrbwbubbruwbb\nuwwwbbggwrgbrgrubrurwrgugrbubuwwruugbwbgubugbuguuuuurbrgr\nrrbubwbuwrgrrugubbbuuuwwbwgurrwwgwburubwrwrb\nrurrbbgurbuuruwuuwrurrwbbggrrrgguwgwrurgrurubwrwwrb\nugbugurrgggrgrbuuwgbuugrrgbuuwugbrwrrgbubbbbburuuuwww\nwuwgugruburwguwrwgwbwrbubbrbgwbrgbwruruwbbuwwwugurwgurwrbbb\nwugwbruwuggrruggrbgrgubuubgurbrrrruwrguububruubwugwwbbwbu\ngrubuwwurrbbggwbwwwruuuuubwgwubwuubuuwrrrwgrururbggbbggw\ngwgrwbuwuwgwrubbgbugrgwbgrbwbuwgrggbwrrubbuggwbgrwgbggg\nuruwrwuwbrbrwwruwgurrugrbwguuubwrwwurubgrbgrgwwur\nrguubrwwgubuwwruruwbuggbrburgrgurugwwwwrb\nuuubuubggrugbgbgwgbbgburuwggrrggwrwruwgbuwwbrgu\ngwgrgugwgbwbuwbgwgbrguuguguugrrgrbuugugbrgu\nurgrwwwrgurwwrwwwggbgubbrgwwwruwubgbrgurguurwugrgwrb\nrubgwbrwbgrruuwbruwrgwbwbguwururubrgwrurbuubww\nbrurbguurgbggwbbgwwwugbrbgwrwbrwrrbrwbugwuguwrbwru\nrwrbbguggugwwgrbrrwrbgruwrwwuugbrgurbwuguwwubgbgg\nwgrgbgbwbbggrwgrbbbrrwubgrbrbgwwururguwugbgrgrrug\ngwuurwubwwguggwwbbwwugrwgggwwurrrgrrrburguwwrrb\nguggrruwrbrugwrwgrbgurbgbrgwugwwwwbbbwwrwuwug\nuwgrrgrbbgwrggrwwwgbgbrbbrbuuburbbrbrugwurugwbburgbb\nwwwbbbwbbbrbgubrwbbrubugbrgrrrruuwgurrwwwruwgwrguw\nuuubuwgwrwugrbggggbruugbrruwuurubwwgwbwgurbgbuubbgwbuww\nwbrrwgbuwggubuggrugbwwbbbbwgwrrbgggrrrwrbgrbgg\ngbbbrwwggbugrbrrwrgbuwgbrrrwgwgubrruruurwguwb\nrrbbuwrbruwruwurbggburwwbwuuwrurbbwrbuurubggwrb\nrrubbuurrrgbrwwuwrbwgruuwbbwugrgubgbwwruwbburgbwb\nwrwugbbgrbgurubrwwwwwbbbruubwgrgburbwbrgbwbgwb\nwwrwugwbbrubugbrrgrwwbwbuwwwuugbbwguruggwgwrwgwrggwrgrgwgwrb\nbguwgugwbgwgubwwbwwrwubrrwubbwgrbwgggwuuwgrbgwgwgrwwggrb"
  out "Answer":u32
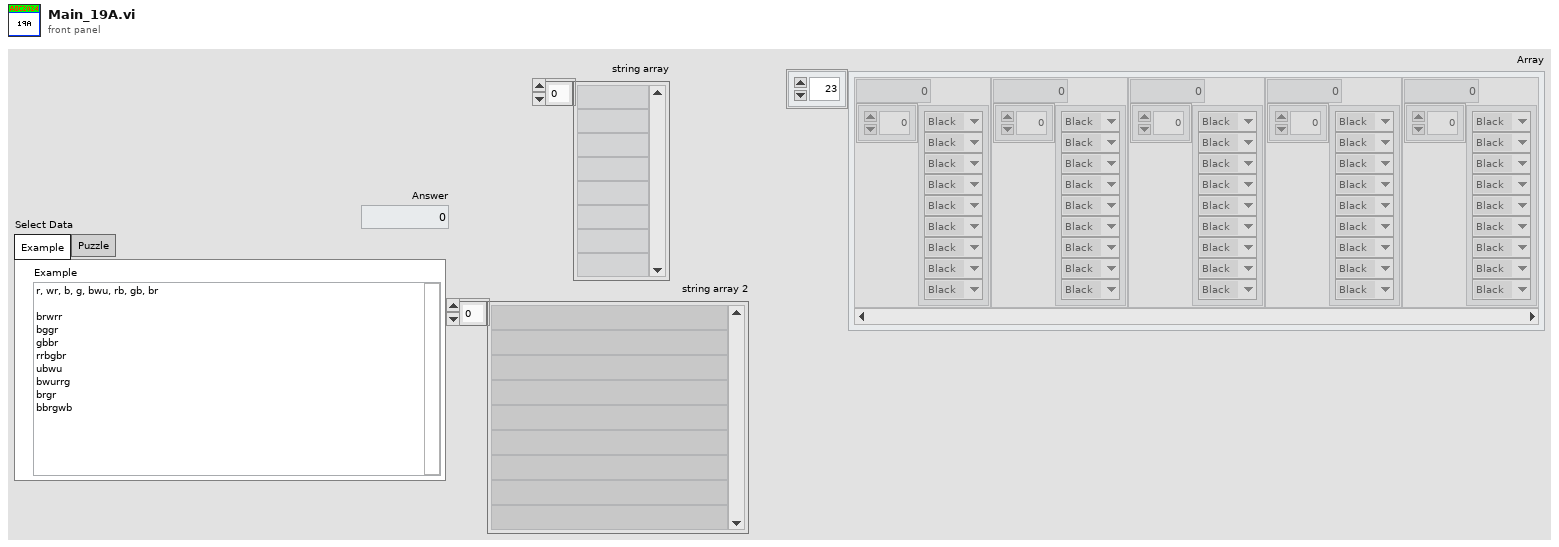
[diagram p1: front panel]
types:
  T1 = typedef "ENUM_Stripe Select.ctl" = enum16{"Black", "Blue", "Green", "Red", "White"}
  T2 = typedef "ENUM_8 Directions U-D-L-R.ctl" = enum16{"Up;-1,0", "Up-Right;-1,1", "Right;0,1", "Down-Right;1,1", "Down;1,0", "Down-Left;1,-1", "Left;0,-1", "Up-Left;-1,-1"}
  T3 = typedef "ENUM_4 Directions U-D-L-R.ctl" = enum16{"Up;-1,0", "Right;0,1", "Down;1,0", "Left;0,-1"}
  T4 = typedef "Cluster_Row-Column.ctl" = cluster{"R":i32, "C":i32}
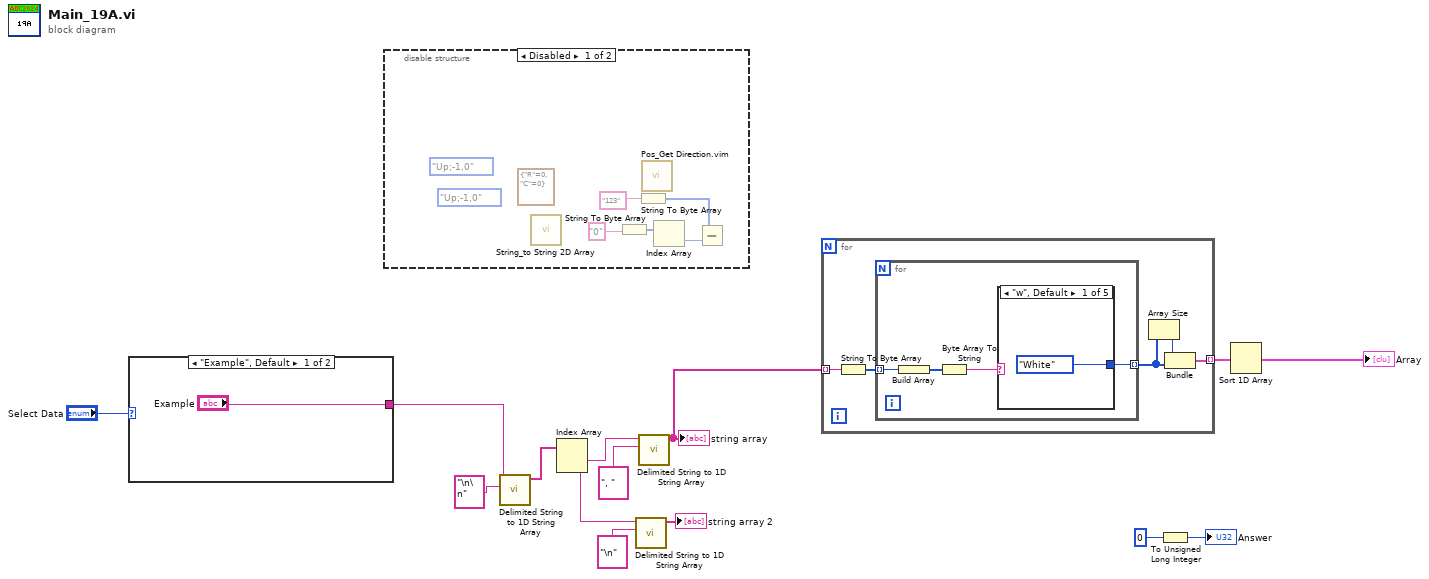
[diagram p0: block diagram]
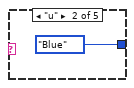
[diagram p2: hidden frame]
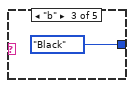
[diagram p3: hidden frame]
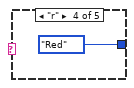
[diagram p4: hidden frame]
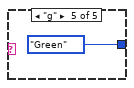
[diagram p5: hidden frame]
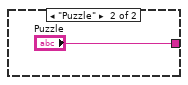
[diagram p6: hidden frame]
diagram:
  n1 = case shown="\"Example\", Default" "Select Data" {
    tunnel: ["Example" "Puzzle"] -> w10
    frame "Example", Default {
    }
    frame "Puzzle" {
    }
  }
  n2 = disable-structure shown="Disabled" {
    frame Disabled {
      (unwired) ENUM_8_Directions_U-D-L-R."Up;-1,0" ("Direction 8")
      (unwired) ENUM_4_Directions_U-D-L-R."Up;-1,0" ("Direction")
      (unwired) T4 {"R"=0, "C"=0} ("Position")
      n3 = call "String_to String 2D Array.vi"() -> ()  [unwired: 11 in, 1 out]
      n4 = String To Byte Array(string="0") -> (unsigned byte array=w19:u8[])
      n5 = String To Byte Array(string="123") -> (unsigned byte array=w17:u8[])
      n6 = call "Pos_Get Direction.vim"() -> ()  [unwired: 11 in, 1 out]
      n7 = Index Array(array=w19) -> (element=w18:u8)  [unwired: 1 in]
      n8 = Subtract(x=w17, y=w18) -> ()  [unwired: 1 out]
    }
    frame Enabled {
    }
  }
  n9 = call <vilib>:"Delimited String to 1D String Array.vi"("delimiter"="\n\n" ("delimiter (Tab)"), "delimited string"=w10) -> ("string array"=w9:string[])  [unwired: 9 in]
  n10 = Index Array(array=w9) -> (element #1=w8:string, element #2=w6:string)  [unwired: 2 in]
  n11 = call <vilib>:"Delimited String to 1D String Array.vi"("delimiter"="\n" ("delimiter (Tab)"), "delimited string"=w6) -> ("string array"=→"string array 2":string[])  [unwired: 9 in]
  n12 = call <vilib>:"Delimited String to 1D String Array.vi"("delimiter"=", " ("delimiter (Tab)"), "delimited string"=w8) -> ("string array"=w3:string[])  [unwired: 9 in]
  "string array" <- w3
  n13 = for {
    tunnel: w3 -> [w25] mode=indexing
    tunnel: [w22] -> w2 mode=indexing
    n14 = String To Byte Array(string=w25) -> (unsigned byte array=w26:u8[])
    n15 = for {
      tunnel: w26 -> [w30] mode=indexing
      tunnel: [w27] -> w23 mode=indexing
      n16 = Build Array(w30) -> (w29:u8[])
      n17 = Byte Array To String(unsigned byte array=w29) -> (string=w28:string)
      n18 = case shown="\"w\", Default" w28 {
        tunnel: [ENUM_Stripe_Select."White" ("Stripe Select") ENUM_Stripe_Select."Blue" ("Stripe Select") ENUM_Stripe_Select."Black" ("Stripe Select") ENUM_Stripe_Select."Red" ("Stripe Select") ENUM_Stripe_Select."Green" ("Stripe Select")] -> w27
        frame "w", Default {
        }
        frame "u" {
        }
        frame "b" {
        }
        frame "r" {
        }
        frame "g" {
        }
      }
    }
    n19 = Array Size(array=w23) -> (size(s)=w24:i32)
    n20 = Bundle(w24, w23) -> (w22:cluster{i32, T1[]})  [unwired: 1 in]
  }
  n21 = To Unsigned Long Integer(number=u32 0) -> (unsigned 32bit integer=→"Answer":u32)
  n22 = Sort 1D Array(array=w2) -> (sorted array=→"Array":cluster{i32, T1[]}[])
